vi "Collect UI Refs.vi"(8 "error in (no error)":errorcluster, 9 "Container":refnum<vi>, 10 "Layout Panel VI":refnum<vi>, 11 "2DArrayManager in":refnum<class "2DArrayManager.lvclass">) -> (0 "error out":errorcluster, 3 "2DArrayManager out":refnum<class "2DArrayManager.lvclass">)   [LabVIEW 2020, in "OOPanel.lvlib" / "2DArrayManager.lvclass"]
uses:
  2DArrayManager.lvclass
  UI Refs.ctl
  2DPanelBlank/2DPanelBlank.lvclass
panel:
  out "Array":string[](array[string])
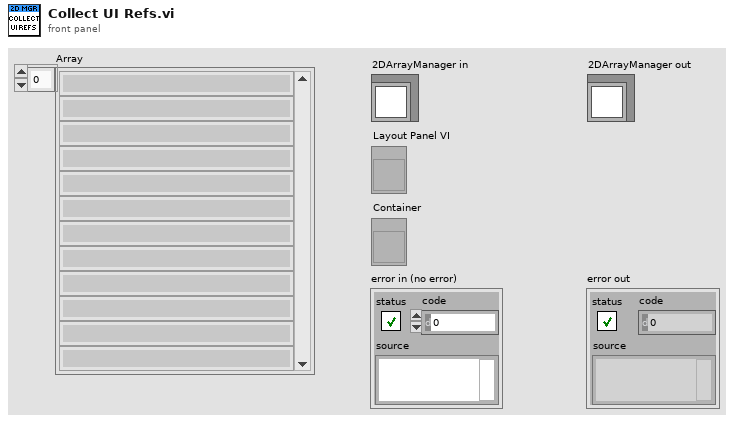
[diagram p1: front panel]
types:
  T1 = typedef "OOPanel.lvlib/2DArrayManager.lvclass/UI Refs.ctl" = cluster{"Panel VI":refnum<vi>, "Container":refnum<vi>, "H Scroll":refnum<vi>, "V Scroll":refnum<vi>, "Owning VI":refnum<vi>, "FP":refnum<vi>, "Corner":refnum<vi>, "Used Panels":set{refnum<vi>}, "Blank Pool":refnum<queue>, "Blank":refnum<class "2DPanelBlank.lvclass">, "Use Blank":bool, "Used Blanks":set{refnum<class "2DPanelBlank.lvclass">}}
  T2 = typedef "OOPanel.lvlib/2DArrayManager.lvclass/State.ctl" = cluster{"Scroll":T3, "Scroll Max":T3, "Top-Left Index":T4, "H Scroll Sync":refnum<user-event>, "V Scroll Sync":refnum<user-event>, "Sync":bool, "H Scroll Vis":bool, "V Scroll Vis":bool, "Blank Pool":refnum<queue>}
  T3 = typedef "OOPanel.lvlib/2D Position.ctl" = cluster{"H":i32, "V":i32}
  T4 = typedef "OOPanel.lvlib/2D Index.ctl" = cluster{"Row":i32, "Col":i32}
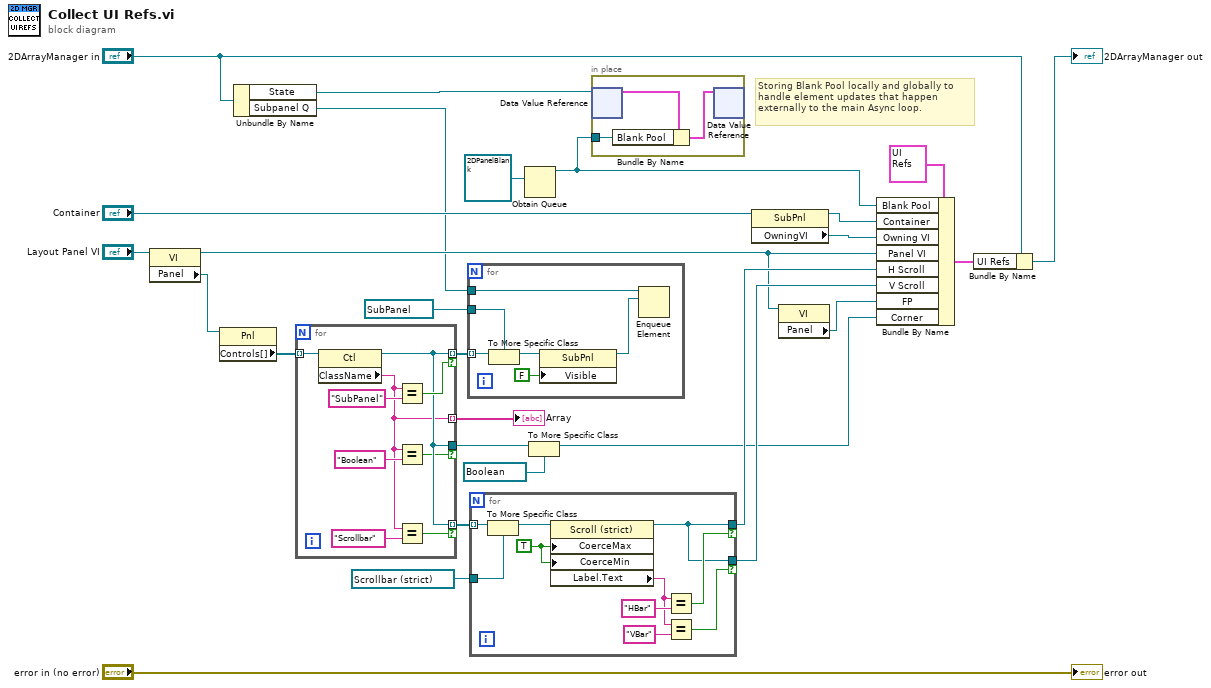
[diagram p0: block diagram]
diagram:
  # "Storing Blank Pool locally and globally to handle element updates that happen externally to the main Async loop."
  n1 = property class="VI"(reference="Layout Panel VI") -> (reference out=w13:refnum<vi>, "Panel"=w26:refnum<vi>)  [unwired: 1 in, 1 out]
  n2 = property class="Pnl"(reference=w26) -> ("Controls[]"=w23:refnum<vi>[])  [unwired: 1 in, 2 out]
  n3 = Unbundle By Name("2DArrayManager in") -> ("State"=w5:refnum<data-value>, "Subpanel Q"=w1:refnum<queue>)
  n4 = for {
    tunnel: w23 -> [w36] mode=indexing
    tunnel: [w30] -> w22 mode=indexing if=w34
    tunnel: [w30] -> w25 mode=indexing if=w32
    tunnel: [w30] -> w10 if=w29
    tunnel: [w28] -> w11 mode=indexing
    n5 = property class="Ctl"(reference=w36) -> (reference out=w30:refnum<vi>, "ClassName"=w28:string)  [unwired: 1 in, 1 out]
    n6 = Equal?(x=w28, y="SubPanel") -> (x = y?=w34:bool)
    n7 = Equal?(x=w28, y="Boolean") -> (x = y?=w29:bool)
    n8 = Equal?(x=w28, y="Scrollbar") -> (x = y?=w32:bool)
  }
  "Array" <- w11
  n9 = for {
    tunnel: refnum<vi> refnum ("target class") -> [w40]
    tunnel: w22 -> [w39] mode=indexing
    tunnel: w1 -> [w37]
    n10 = To More Specific Class(target class=w40, reference=w39) -> (specific class reference=w42:refnum<vi>)  [unwired: 1 in, 1 out]
    n11 = property class="SubPnl"(reference=w42, "Visible"=FALSE) -> (reference out=w38:refnum<vi>)  [unwired: 1 in, 1 out]
    n12 = Enqueue Element(queue=w37, element=w38) -> ()  [unwired: 2 in, 3 out]
  }
  n13 = for {
    tunnel: w25 -> [w52] mode=indexing
    tunnel: refnum<vi> refnum ("Scrollbar") -> [w51]
    tunnel: [w44] -> w17 if=w45
    tunnel: [w44] -> w16 if=w43
    w49 = TRUE ("Coerce Maximum Value")
    n14 = To More Specific Class(target class=w51, reference=w52) -> (specific class reference=w50:refnum<vi>)  [unwired: 1 in, 1 out]
    n15 = property class="Scroll (strict)"(reference=w50, "CoerceMax"=w49, "CoerceMin"=w49) -> (reference out=w44:refnum<vi>, "Label.Text"=w46:string)  [unwired: 1 in, 1 out]
    n16 = Equal?(x=w46, y="HBar") -> (x = y?=w45:bool)
    n17 = Equal?(x=w46, y="VBar") -> (x = y?=w43:bool)
  }
  n18 = Obtain Queue(element data type=refnum<class "2DPanelBlank.lvclass"> refnum ("OOPanel.lvlib:2DPanelBlank.lvclass")) -> (queue out=w3:refnum<queue>)  [unwired: 4 in, 2 out]
  n19 = To More Specific Class(target class=refnum<vi> refnum, reference=w10) -> (specific class reference=w8:refnum<vi>)  [unwired: 1 in, 1 out]
  n20 = in-place {
    in-place-border: w3 -> [w53]
    n21 = in-place-dvr #1(w5) -> (w55:T2)  [unwired: 1 out]
    n22 = Bundle By Name(cluster=w55, "Blank Pool"=w53) -> (w54:T2)
    n23 = in-place-dvr #1(w54) -> ()  [unwired: 2 out]
  }
  n24 = property class="SubPnl"(reference="Container") -> (reference out=w19:refnum<vi>, "OwningVI"=w18:refnum<vi>)  [unwired: 1 in, 1 out]
  n25 = property class="VI"(reference=w13) -> ("Panel"=w12:refnum<vi>)  [unwired: 1 in, 2 out]
  n26 = Bundle By Name(cluster=T1 {"Panel VI"=refnum, "Container"=refnum, "H Scroll"=refnum, "V Scroll"=refnum, "Owning VI"=refnum, "FP"=refnum, "Corner"=refnum, "Used Panels"={}, "Blank Pool"=refnum, "Blank"=refnum, "Use Blank"=FALSE, "Used Blanks"={}} ("UI Refs"), "Blank Pool"=w3, "Container"=w19, "Owning VI"=w18, "Panel VI"=w13, "H Scroll"=w17, "V Scroll"=w16, "FP"=w12, "Corner"=w8) -> (w7:T1)
  n27 = Bundle By Name(cluster="2DArrayManager in", "UI Refs"=w7) -> (→"2DArrayManager out":refnum<class "2DArrayManager.lvclass">)
  "error out" <- "error in (no error)"
